vi "counterTool_23_S_inc_enc.vi"(0 "Counts":dbl, 2 "Zero":bool, 3 "Couts/rev":dbl=7408.8, 4 "Output Units":enum16{"Degrees", "Radians"}(ring)) -> (6 "Total Angle":dbl=72.0, 7 "Wrap Angle":dbl)   [LabVIEW 2023]
doc: "Voltage - Input voltage value\nDeg/Volt - Constant multiplier to convert input voltage to angular value\n\nTotal Angle - Current accumulated angle -Inf to Inf degrees\nWrap Angle - Current angle 0 to 360 degrees"
panel:
  in  "zer":dbl
  out "Cycles":dbl
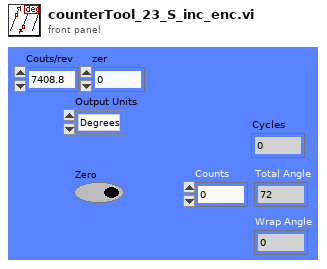
[diagram p1: front panel]
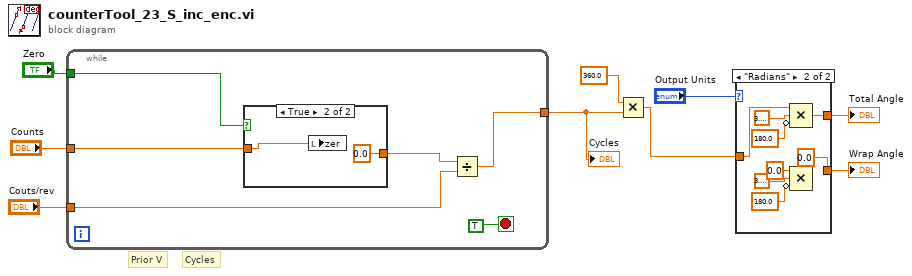
[diagram p0: block diagram]
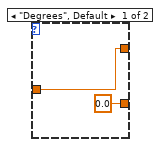
[diagram p2: hidden frame]
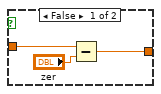
[diagram p3: hidden frame]
diagram:
  # "Prior V"
  # "Cycles"
  n1 = while {
    tunnel: "Counts" -> [w13]
    tunnel: "Zero" -> [w14]
    tunnel: "Couts/rev" -> [w11]
    tunnel: [w10] -> w1
    stop <- TRUE stop-if-true
    n2 = case shown="True" w14 {
      tunnel: w13 -> [w18 w20]
      tunnel: [w16 0.0] -> w12
      frame False {
        n3 = Subtract(x=w18, y="zer") -> (x-y=w16:dbl)
      }
      frame True {
        n4 = local write "zer"(w20) -> ()
      }
    }
    n5 = Divide(x=w12, y=w11) -> (x/y=w10:dbl)
  }
  "Cycles" <- w1
  n6 = Multiply(x=360.0 ("y"), y=w1) -> (x*y=w9:dbl)
  n7 = case shown="\"Radians\"" "Output Units" {
    tunnel: [w22 w28] -> w4
    tunnel: w9 -> [w22 w27]
    tunnel: [0.0 0.0] -> w3
    frame "Degrees", Default {
    }
    frame "Radians" {
      n8 = Compound Arithmetic op=MULTIPLY(w27, 3.141592653589793, invert 180.0 ("value")) -> (w28:dbl)
      n9 = Compound Arithmetic op=MULTIPLY(0.0 ("value"), 3.141592653589793, invert 180.0 ("value")) -> ()  [unwired: 1 out]
    }
  }
  "Wrap Angle" <- w3
  "Total Angle" <- w4
